vi "ClearOldNodeHTMLFiles.vi"(3 "ROS":T1={"topic port"=7000, "Node"="/LVROS", "topic"="/LVROS", "type"="", "node port"=7000, "error "={"status"=FALSE, "code"=0, "source"=""}, "Direction"=enum."Node", "Update (ms)"=1, "FIFO size"=1}) -> (1 "ROS out":T1={"topic port"=7000, "Node"="/LVROS", "topic"="/LVROS", "type"="", "node port"=7000, "error "={"status"=FALSE, "code"=0, "source"=""}, "Direction"=enum."Node", "Update (ms)"=1, "FIFO size"=1})   [LabVIEW 2014]
doc: "Deletes old HTML files for unused nodes"
uses:
  <userlib>/ROS for LabVIEW Software.lnk/ROS/Code/SubVIs/_ROSControl.ctl
  <userlib>/ROS for LabVIEW Software.lnk/ROS/Code/SubVIs/_ROSDirection.ctl
panel:
  out "Files deleted":string[](array[string])
  out "filenames":string[](array[string])
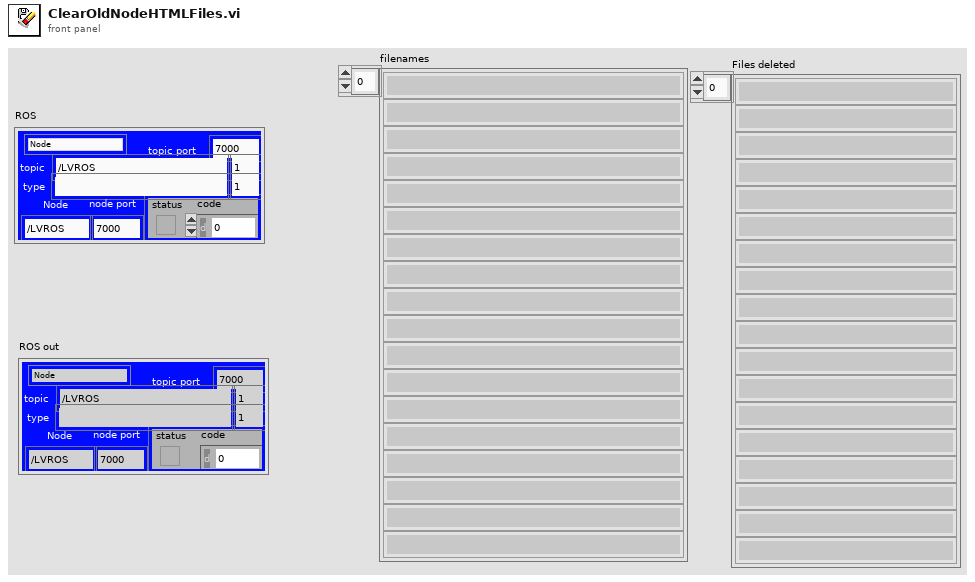
[diagram p1: front panel]
types:
  T1 = typedef "_ROSControl.ctl" = cluster{"topic port":u16, "Node":string, "topic":string, "type":string, "node port":u16, "error ":errorcluster, "Direction":T2, "Update (ms)":u16, "FIFO size":u16}
  T2 = typedef "_ROSDirection.ctl" = enum16{"Node", "Publisher", "Subscriber", "ServiceClient", "ServiceProvider"}
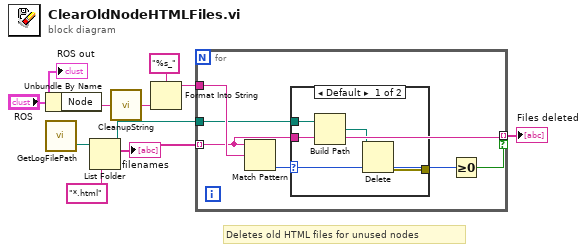
[diagram p0: block diagram]
diagram:
  # "Deletes old HTML files for unused nodes"
  n1 = Unbundle By Name("ROS") -> ("Node"=w4:string)
  n2 = call <userlib>:"GetLogFilePath.vi"() -> ("LogFolder"=w9:path)  [unwired: 2 in, 1 out]
  n3 = List Folder(path=w9, pattern="*.html") -> (path out=w5:path, filenames=w7:string[])  [unwired: 2 in, 2 out]
  "filenames" <- w7
  n4 = call <userlib>:"CleanupString.vi"("String"=w4) -> ("url"=w3:string)
  n5 = Format Into String(format string="%s_", w3) -> (resulting string=w6:string)  [unwired: 2 in, 1 out]
  n6 = for {
    tunnel: w7 -> [w13] mode=indexing
    tunnel: w6 -> [w15]
    tunnel: w5 -> [w14]
    tunnel: [w13] -> w2 mode=indexing if=w11
    n7 = Match Pattern(string=w13, regular expression=w15) -> (offset past match=w12:i32)  [unwired: 1 in, 3 out]
    n8 = case shown="Default" w12 {
      tunnel: w14 -> [w19 _]
      tunnel: w13 -> [w18 _]
      tunnel: [w16 _] -> _
      frame Default {
        n9 = Build Path(base path=w19, name or relative path=w18) -> (appended path=w17:path)
        n10 = Delete(path (use dialog)=w17) -> (error out=w16:errorcluster)  [unwired: 4 in, 2 out]
      }
      frame -1 {
      }
    }
    n11 = Greater Or Equal To 0?(x=w12) -> (x >= 0?=w11:bool)
  }
  "Files deleted" <- w2
  "ROS out" <- "ROS"
